vi "Set Delete User.vi"(7 "User Index":i32, 8 "error IO":errorcluster, 11 "VISA resource name":refnum<visa-resource-name>) -> (0 "error Out":errorcluster, 3 "VISA resource Out":refnum<visa-resource-name>)   [LabVIEW 2020, in "Associated Research 78XX Series.lvlib"]
uses:
  <instrlib>/Associated Research 78XX Series/Associated Research 78XX Series.lvlib
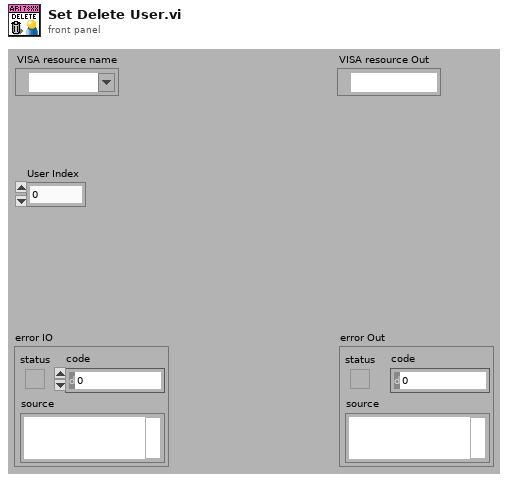
[diagram p1: front panel]
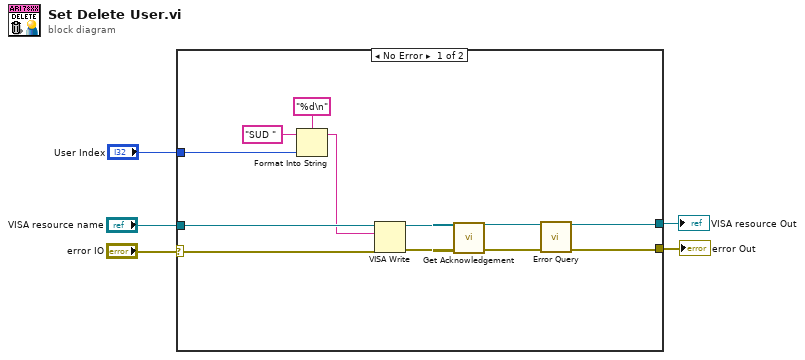
[diagram p0: block diagram]
diagram:
  n1 = case shown="No Error" "error IO" {
    selector: "error IO" -> [w14 w19]
    tunnel: [w16 w19] -> w2
    tunnel: [w17 w18] -> w3
    tunnel: "VISA resource name" -> [w13 w18]
    tunnel: "User Index" -> [w15 _]
    frame No Error {
      n2 = Format Into String(format string="%d\n", initial string="SUD " ("Command to Send (empty)"), w15) -> (resulting string=w8:string)  [unwired: 1 in, 1 out]
      n3 = VISA Write(VISA resource name=w13, write buffer=w8, error in (no error)=w14) -> (VISA resource name out=w6:refnum<visa-resource-name>, error out=w7:errorcluster)  [unwired: 1 out]
      n4 = call <instrlib>:"Get Acknowledgement.vi"("VISA resource name"=w6, "error in (no error)"=w7) -> ("VISA resource name out"=w11:refnum<visa-resource-name>, "error out"=w12:errorcluster)  [unwired: 12 in]
      n5 = call <instrlib>:"Error Query.vi"("VISA resource name"=w11, "error in (no error)"=w12) -> ("VISA resource name out"=w17:refnum<visa-resource-name>, "error out"=w16:errorcluster)  [unwired: 10 in, 2 out]
    }
    frame Error {
    }
  }
  "VISA resource Out" <- w3
  "error Out" <- w2
